vi "获取128X4频率.vi"(6 "testType":string, 7 "ref":bool=TRUE, 8 "error in (no error)":errorcluster, 9 "COM":i32, 11 "A":i32) -> (0 "error out":errorcluster, 2 "Freq&S21":string[][](table))   [LabVIEW 2015]
uses:
  Database_util/Ctl/database_Method.ctl
  network_Global/Global.vi
panel:
  out "搜索结果":i32
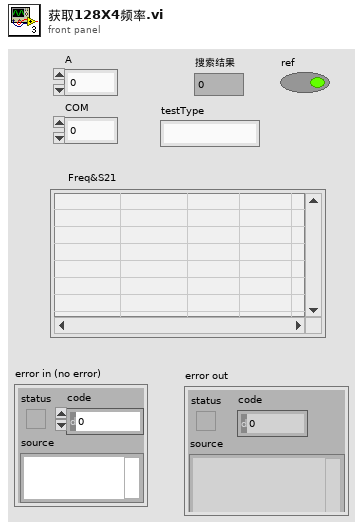
[diagram p1: front panel]
types:
  T1 = typedef "database_Method.ctl" = enum16{"初始化", "查询", "关闭"}
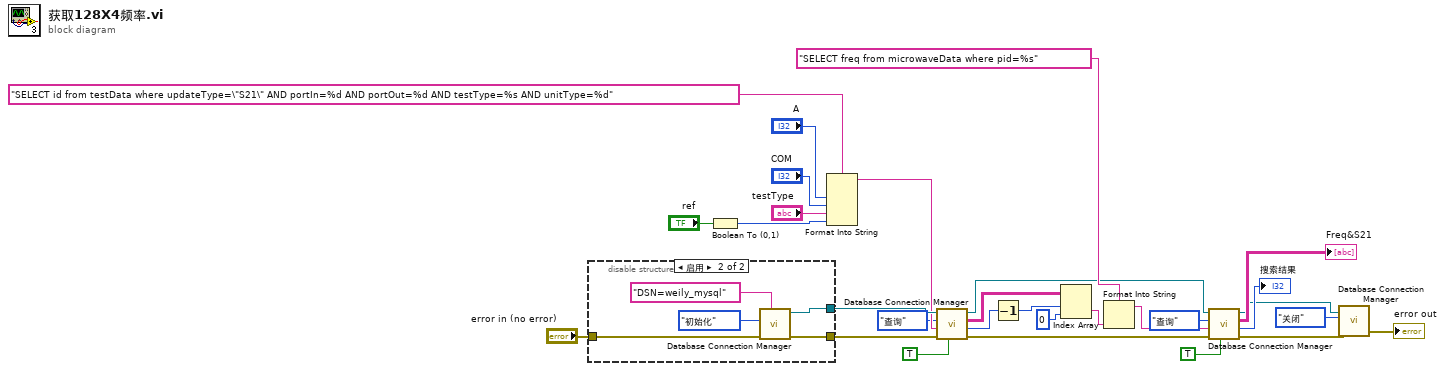
[diagram p0: block diagram]
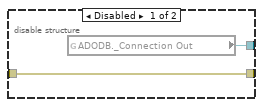
[diagram p2: hidden frame]
diagram:
  n1 = disable-structure shown="启用" {
    disable-tunnel: [w31 w34] -> w20
    disable-tunnel: "error in (no error)" -> [w30 w33]
    disable-tunnel: [w30 w32] -> w9
    frame Disabled {
      n2 = global read "Global.vi" "ADODB._Connection Out"() -> (w31:refnum<k7>)
    }
    frame Enabled {
      n3 = call "Database Connection Manager.vi"("ConnectionString"="DSN=weily_mysql", "error in (no error)"=w33, "Method"=database_Method."初始化") -> ("error out"=w32:errorcluster, "ADODB._Connection Out"=w34:refnum<k7>)  [unwired: 5 in, 2 out]
    }
  }
  n4 = Boolean To (0,1)(Boolean="ref") -> (0, 1=w7:i16)
  n5 = Format Into String(format string="SELECT id from testData where updateType=\"S21\" AND portIn=%d AND portOut=%d AND testType=%s AND unitType=%d" ("SQL"), "A", "COM", "testType", w7) -> (resulting string=w19:string)  [unwired: 2 in, 1 out]
  n6 = call "Database Connection Manager.vi"("Return Data (T)"=TRUE, "error in (no error)"=w9, "Command Text"=w19, "Method"=database_Method."查询", "ADODB._Connection In"=w20) -> ("error out"=w16:errorcluster, "Rows Fetched"=w17:i32, "Data"=w18:string[][], "ADODB._Connection Out"=w15:refnum<k7>)  [unwired: 3 in]
  n7 = Decrement(x=w17) -> (x-1=w28:i32)
  n8 = Index Array(array=w18, index (row)=w28, index (col)=0 ("disabled index (col)")) -> (element=w26:string)
  n9 = Format Into String(format string="SELECT freq from microwaveData where pid=%s" ("String"), w26) -> (resulting string=w14:string)  [unwired: 2 in, 1 out]
  n10 = call "Database Connection Manager.vi"("Return Data (T)"=TRUE, "error in (no error)"=w16, "Command Text"=w14, "Method"=database_Method."查询", "ADODB._Connection In"=w15) -> ("error out"=w2:errorcluster, "Rows Fetched"=→"搜索结果":i32, "Data"=→"Freq&S21":string[][], "ADODB._Connection Out"=w3:refnum<k7>)  [unwired: 3 in]
  n11 = call "Database Connection Manager.vi"("error in (no error)"=w2, "Method"=database_Method."关闭", "ADODB._Connection In"=w3) -> ("error out"=→"error out":errorcluster)  [unwired: 5 in, 3 out]
